vi "Old_OptimizationFunction.vi"(9 "output selector":T1, 10 "data":variant, 11 "Input parameters":dbl[](array[numeric])=[8.0, -2.0, 0.02] step=1e-10 format="%#.8f") -> (0 "error out":errorcluster, 1 "Inequality Constraints":dbl[](array[numeric]), 2 "Equality Constraints":dbl[](array[numeric]), 3 "Mean squared error":dbl)   [LabVIEW 2020]
uses:
  <vilib>/gmath/NumericalOptimization/cno_output select.ctl
  Camera software flag.vi
  Global line error.vi
  <vilib>/gmath/NI_Gmath.lvlib
panel:
  out "Global line error 2":dbl=4.855450477427298
  out "Global line error":dbl=4.85465868905039
  in  "Goal function from 10fps":dbl[](array[numeric])=[-0.4027, 0.9312, -0.0635, -0.0114] step=1e-10 format="%#.8f"
  in  "Save input parameter history":path
  in  "Save input parameters to file":bool
  in  "Goal function from 1fps":dbl[](array[numeric])=[-0.4089, 0.8704, -0.0731, -0.0215] step=1e-10 format="%#.8f"
  in  "Flyback time (ms)":dbl
  in  "Acquisition time (ms)":dbl=1000.0
  in  "X":dbl[](array[numeric])
  in  "Goal function":dbl[](array[numeric])=[-0.407, 0.781, 0.00845, -0.0056] step=1e-10 format="%#.8f"
  # "A*t^3+B*t^2+C*t+D"
  # "-0.249910;0.582909;-0.041239;-0.005871"
  # "D"
  # "C"
  # "B"
  # "A"
  # "-0.239308;0.566047;-0.039762;-0.004251"
  # "-0.235642;0.577058;-0.040959;-0.006304"
  # "-0.241529;0.576644;-0.050284;-0.005285"
  # "-0.236851;0.564288;-0.038353;-0.007365"
  # "-0.239346;0.590340;-0.053160;-0.004322"
  # "D"
  # "-0.230329;0.601481;-0.025737;-0.004707"
  # "C"
  # "A*t^3+B*t^2+C*t+D"
  # "Goal function from 1Hz"
  # "y = -0.0215x3 - 0.0731x2 + 0.8704x - 0.4089"
  # "B"
  # "A"
  # "y = -0.0114x3 - 0.0635x2 + 0.9312x - 0.4027"
  # "Goal function from 5Hz frame 143"
  # "y = -5.1846x3 - 1.8975x2 + 4.5313x - 0.4041"
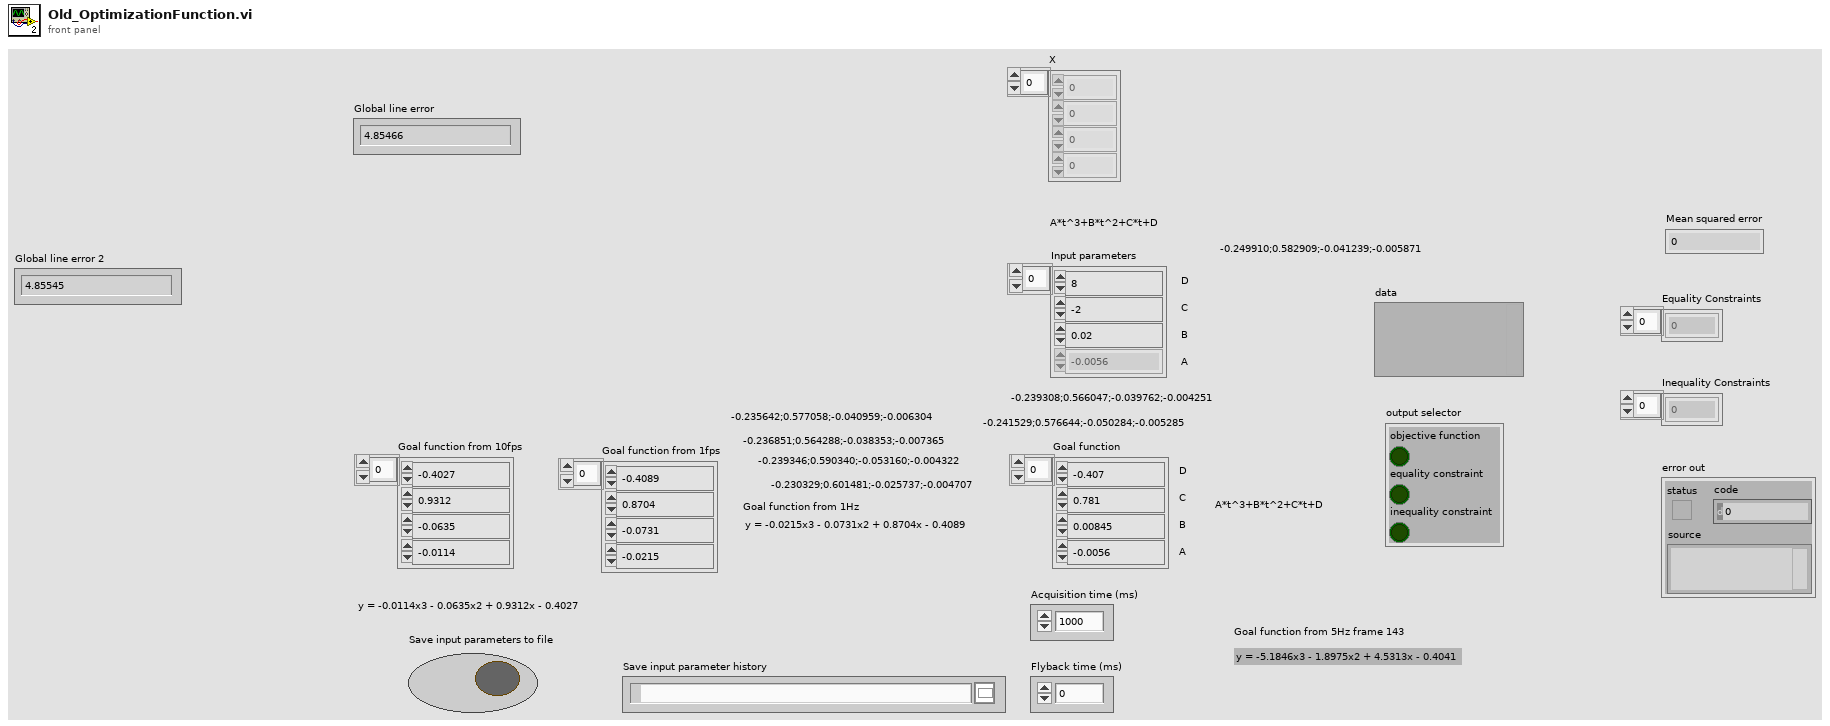
[diagram p1: front panel]
types:
  T1 = typedef "NI_Gmath.lvlib/cno_output select.ctl" = cluster{"objective function":bool, "equality constraint":bool, "inequality constraint":bool}
  T2 = enum16{"open", "replace", "create", "open or create", "replace or create", "replace or create with confirmation"}
  T3 = cluster{"Input parameters[0]":dbl, "Input parameters[1]":dbl, "Input parameters[2]":dbl, "Input parameters[3]":dbl, "Input parameters[4]":dbl, "Input parameters[5]":dbl, "Input parameters[6]":dbl, "Input parameters[7]":dbl, "Input parameters[8]":dbl}
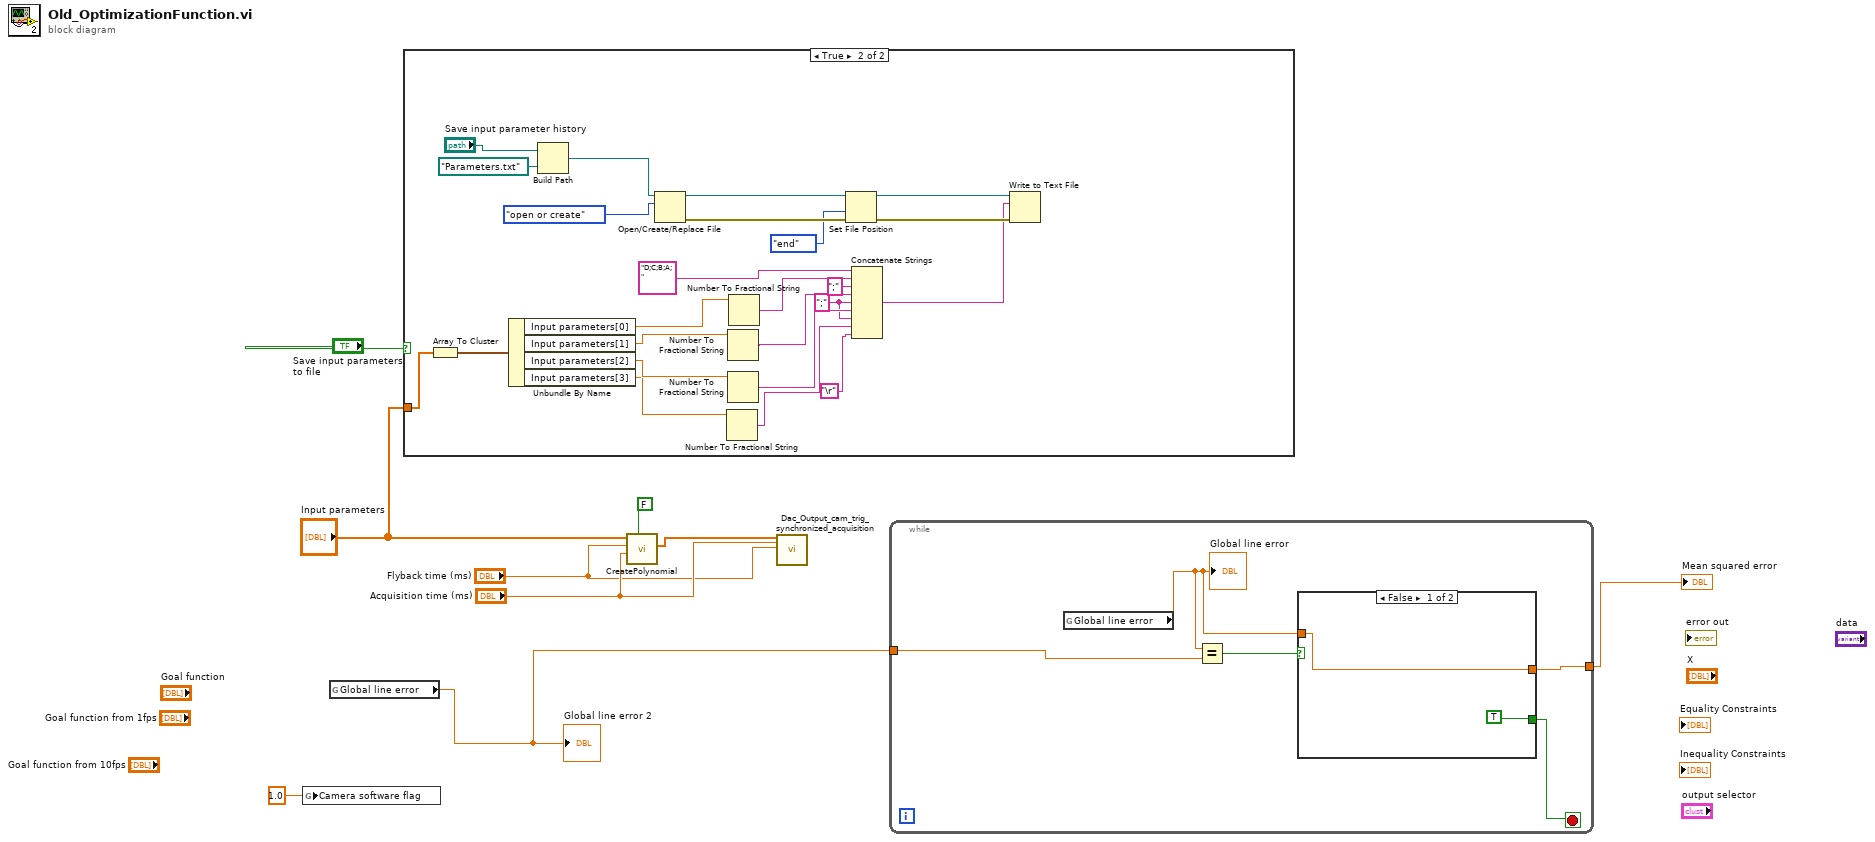
[diagram p0: block diagram]
diagram:
  n1 = global write "Camera software flag.vi" "Camera software flag"(1.0 ("Camera software flag")) -> ()
  n2 = global read "Global line error.vi" "Global line error"() -> (w3:dbl)
  "Global line error 2" <- w3
  n3 = case shown="True" "Save input parameters to file" {
    tunnel: "Input parameters" -> [_ w19]
    frame False {
    }
    frame True {
      w13 = ";" ("string")
      n4 = Array To Cluster(array=w19) -> (cluster=w18:T3)
      n5 = Unbundle By Name(w18) -> ("Input parameters[0]"=w17:dbl, "Input parameters[1]"=w16:dbl, "Input parameters[2]"=w15:dbl, "Input parameters[3]"=w12:dbl)
      n6 = Build Path(base path="Save input parameter history", name or relative path=path "Parameters.txt") -> (appended path=w33:path)
      n7 = Open/Create/Replace File(file path (use dialog)=w33, operation (0:open)=T2."open or create") -> (refnum out=w29:refnum<file>, error out=w30:errorcluster)  [unwired: 4 in, 1 out]
      n8 = Number To Fractional String(number=w12) -> (F-format string=w11:string)  [unwired: 3 in]
      n9 = Number To Fractional String(number=w16) -> (F-format string=w22:string)  [unwired: 3 in]
      n10 = Number To Fractional String(number=w15) -> (F-format string=w21:string)  [unwired: 3 in]
      n11 = Number To Fractional String(number=w17) -> (F-format string=w25:string)  [unwired: 3 in]
      n12 = Set File Position(refnum=w29, from (0:start)=enum16{"start", "end", "current"}."end", error in=w30) -> (refnum out=w31:refnum<file>, error out=w32:errorcluster)  [unwired: 1 in]
      n13 = Concatenate Strings("D;C;B;A;" ("text"), w25, ";" ("string"), w22, w13, w21, w13, w11, "\r") -> (w10:string)
      n14 = Write to Text File(file (use dialog)=w31, text=w10, error in=w32) -> ()  [unwired: 1 in, 3 out]
    }
  }
  n15 = call "CreatePolynomial.vi"("Save calibration"=FALSE, "Acquisition time (ms)"="Acquisition time (ms)", "Flyback (ms)"="Flyback time (ms)", "P(x)"="Input parameters") -> ("Generate two signals"=w4:dbl[])  [unwired: 5 in, 1 out]
  n16 = call "Dac_Output_cam_trig_synchronized_acquisition.vi"("LabVIEW generated Sawtooth input"=w4, "Image acquisition time (ms)"="Acquisition time (ms)", "Delay between frames (ms)"="Flyback time (ms)") -> ()  [unwired: 17 in]
  n17 = while {
    tunnel: w3 -> [w38]
    tunnel: [w35] -> w2
    stop <- w34 stop-if-true
    n18 = global read "Global line error.vi" "Global line error"() -> (w36:dbl)
    "Global line error" <- w36
    n19 = Equal?(x=w36, y=w38) -> (x = y?=w37:bool)
    n20 = case shown="False" w37 {
      tunnel: w36 -> [w40 _]
      tunnel: [w40 _] -> w35
      tunnel: [TRUE _] -> w34
      frame False {
      }
      frame True {
      }
    }
  }
  "Mean squared error" <- w2
